vi "Destroy.vi"(8 "error in (no error)":errorcluster, 11 "NotifierMessenger in":refnum<class "NotifierMessenger.lvclass">) -> (0 "error out":errorcluster)   [LabVIEW 2011, in "Messenging.lvlib" / "NotifierMessenger.lvclass"]
uses:
  NotifierMessenger.lvclass
  NotifierMessenger.lvclass/NotifierMessenger.ctl
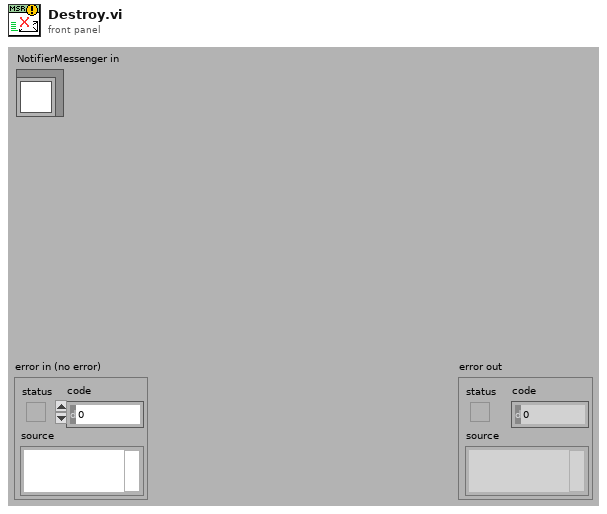
[diagram p1: front panel]
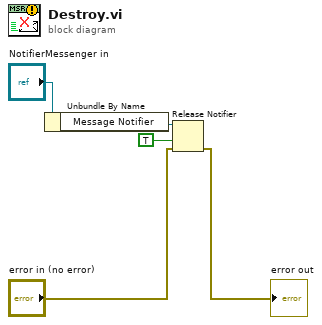
[diagram p0: block diagram]
diagram:
  n1 = Unbundle By Name("NotifierMessenger in") -> ("Message Notifier"=w4:refnum<notifier>)
  n2 = Release Notifier(notifier=w4, force destroy? (F)=TRUE, error in (no error)="error in (no error)") -> (error out=→"error out":errorcluster)  [unwired: 2 out]
